vi "pbcomm32.vi"(1 "error in":errorcluster, 2 "write value":i32 format="%.0x", 3 "address":i16 format="%.0x") -> (0 "error out":errorcluster)   [LabVIEW 2013]
uses:
  WINDOWS/system32/PBD03PC.dll
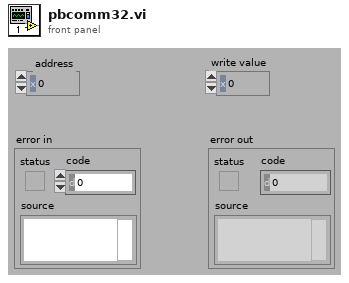
[diagram p1: front panel]
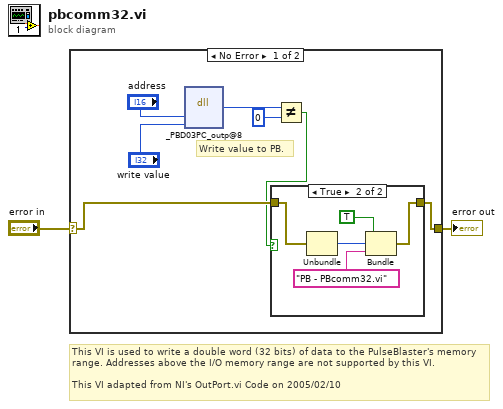
[diagram p0: block diagram]
diagram:
  # "This VI is used to write a double word (32 bits) of data to the PulseBlaster's memory range. Addresses above the I/O memory range are not supported by this VI.\n\nThis VI adapted from NI's OutPort.vi Code on 2005/02/10"
  n1 = case shown="No Error" "error in" {
    selector: "error in" -> [w5 w16]
    tunnel: [w4 w16] -> w2
    frame No Error {
      # "Write value to PB."
      n2 = dll-call lib="C:/WINDOWS/system32/PBD03PC.dll" fn="_PBD03PC_outp@8" label="Call Library Function Node"("address", "write value") -> (w6:i32)  [unwired: 5 in, 2 out]
      n3 = Not Equal?(x=w6, y=0) -> (x != y?=w3:bool)
      n4 = case shown="True" w3 {
        tunnel: w5 -> [w10 w15]
        tunnel: [w10 w14] -> w4
        frame False {
        }
        frame True {
          n5 = Unbundle(w15) -> ("code"=w12:i32)  [unwired: 2 out]
          n6 = Bundle(TRUE, "code"=w12, "PB - PBcomm32.vi") -> (w14:cluster{bool, "code":i32, string})  [unwired: 1 in]
        }
      }
    }
    frame Error {
      # "Error was passed in.\nDo nothing."
    }
  }
  "error out" <- w2
